vi "Vref_NivRef.vi"(10 "Vref":dbl format="%#_13g", 11 "rangosDB in":string[][](array[string])=[["50", "140"], ["40", "130"]]) -> (3 "Vref_NivRef":string[](array[string]))   [LabVIEW 2019, in "Prueba07.lvclass"]
uses:
  Prueba07.lvclass
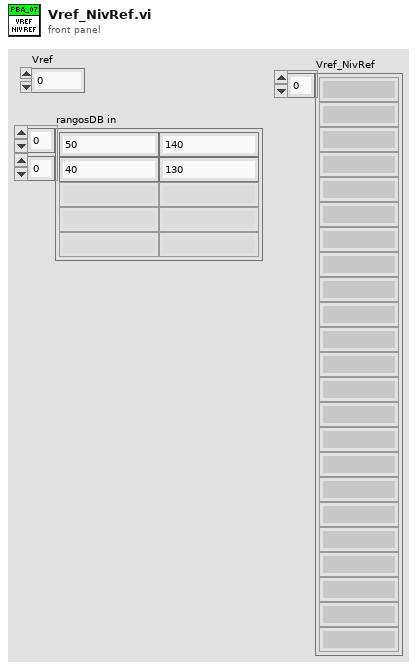
[diagram p1: front panel]
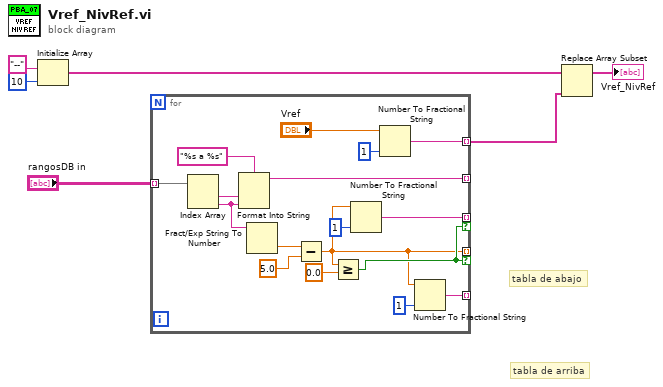
[diagram p0: block diagram]
diagram:
  # "tabla de abajo"
  # "tabla de arriba"
  n1 = Initialize Array("--" ("format string"), 10 ("dimension size")) -> (w3:string[])
  n2 = for {
    tunnel: "rangosDB in" -> [w23] mode=indexing
    tunnel: [w20] -> _ mode=indexing
    tunnel: [w11] -> _ mode=indexing if=w13
    tunnel: [w14] -> _ mode=indexing if=w13
    tunnel: [w10] -> _ mode=indexing
    tunnel: [w7] -> w2 mode=indexing
    n3 = Index Array(array=w23) -> (element #1=w22:string, element #2=w19:string)  [unwired: 2 in]
    n4 = Format Into String(format string="%s a %s", w22, w19) -> (resulting string=w20:string)  [unwired: 2 in, 1 out]
    n5 = Fract/Exp String To Number(string=w19) -> (number=w18:dbl)  [unwired: 3 in, 1 out]
    n6 = Subtract(x=w18, y=5.0) -> (x-y=w11:dbl)
    n7 = Greater Or Equal?(x=w11, y=0.0) -> (x >= y?=w13:bool)
    n8 = Number To Fractional String(number=w11, precision (6)=i16 1) -> (F-format string=w14:string)  [unwired: 2 in]
    n9 = Number To Fractional String(number="Vref", precision (6)=i16 1) -> (F-format string=w7:string)  [unwired: 2 in]
    n10 = Number To Fractional String(number=w11, precision (6)=i16 1) -> (F-format string=w10:string)  [unwired: 2 in]
  }
  n11 = Replace Array Subset(array=w3, new element=w2) -> (→"Vref_NivRef":string[])  [unwired: 1 in]
